vi "MainJSON.vi"(7 "Type and Defaults":variant, 8 "error in":errorcluster, 9 "pathList":string[](array[string])=["$.AnalyticsParameters"], 10 "basePath in":string, 11 "JSON String":string) -> (0 "error out":errorcluster, 1 "Oveerride JSON DATATYPE":T1, 2 "Error Message":string, 3 "VClusterOut":variant)   [LabVIEW 2015, in "Zen Analytics.lvclass"]
doc: "The input array of strings represent the <b>JSON paths</b> to specific elements in the JSON string. These elements are accessed through the path input and the output is provided in the form of <b>VCluster</b> (the bundled form of the input path elements). \nFurthermore, you may use the <b>Variant to Data</b> SubVI to convert back the Variant to the required Cluster type you want."
uses:
  Zen Analytics.lvclass
  Dependency/Override JSON.ctl
  <vilib>/Utility/Data Type/Type Definitions/Data Type.ctl
  <vilib>/regexp/Match Regular Expression.xnode
  <vilib>/addons/_JKI.lib/Serialization/JSON/JKI JSON Serialization.lvlib
  <vilib>/Utility/Data Type/NI_Data Type.lvlib
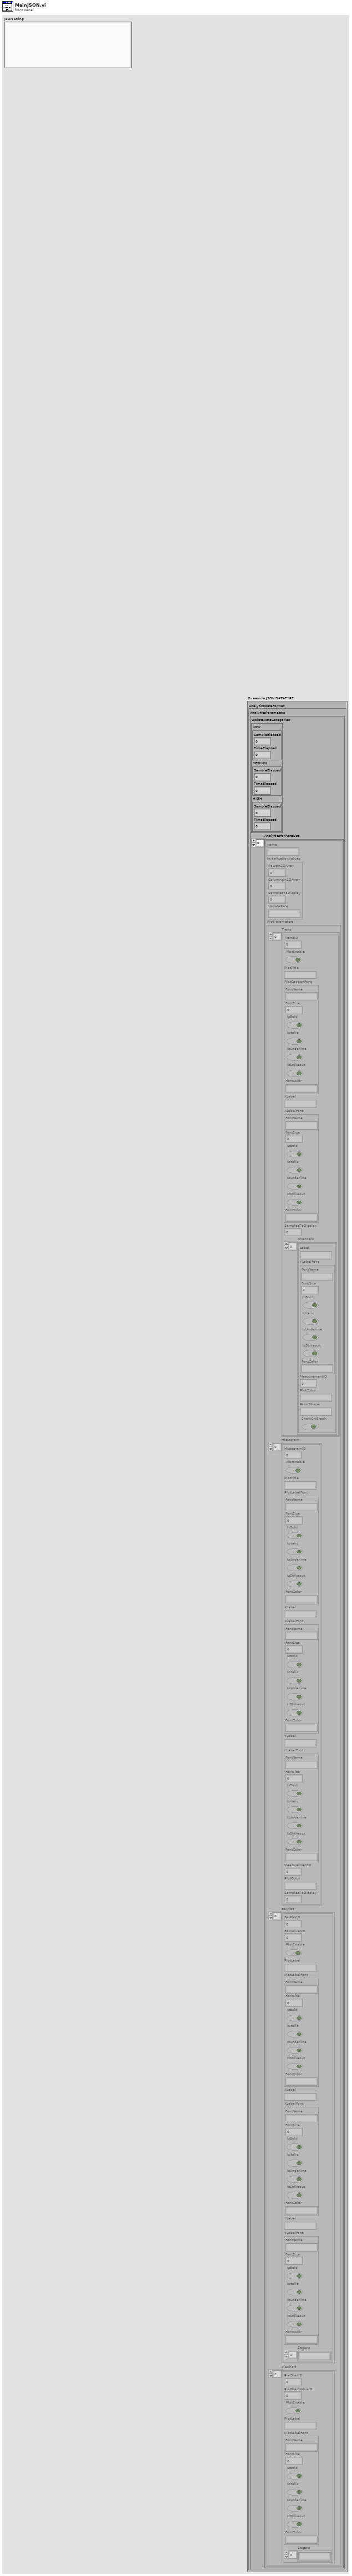
[diagram p1: front panel]
types:
  T1 = typedef "Zen Analytics.lvclass/Override JSON.ctl" = cluster{"AnalyticsDataFormat":cluster{"AnalyticsParameters":cluster{"UpdateRateCategories":cluster{"LOW":cluster{"SampleElapsed":i32, "TimeElapsed":i32}, "MEDIUM":cluster{"SampleElapsed":i32, "TimeElapsed":i32}, "HIGH":cluster{"SampleElapsed":i32, "TimeElapsed":i32}}, "AnalyticsForPartsList":cluster{"Name":string, "InitializationValues":cluster{"RowsIn2DArray":i32, "ColumnsIn2DArray":i32, "SamplesToDisplay":i32, "UpdateRate":string}, "PlotParameters":cluster{"Trend":cluster{"TrendID":i32, "PlotEnable":bool, "PlotTitle":string, "PlotCaptionFont":cluster{"FontName":string, "FontSize":i32, "IsBold":bool, "IsItalic":bool, "IsUnderline":bool, "IsStrikeout":bool, "FontColor":string}, "XLabel":string, "XLabelFont":cluster{"FontName":string, "FontSize":i32, "IsBold":bool, "IsItalic":bool, "IsUnderline":bool, "IsStrikeout":bool, "FontColor":string}, "SamplesToDisplay":i32, "Channels":cluster{"Label":string, "YLabelFont":cluster{"FontName":string, "FontSize":i32, "IsBold":bool, "IsItalic":bool, "IsUnderline":bool, "IsStrikeout":bool, "FontColor":string}, "MeasurementID":i32, "PlotColor":string, "PointShape":string, "ShowOnGraph":bool}[]}[], "Histogram":cluster{"HistogramID":i32, "PlotEnable":bool, "PlotTitle":string, "PlotLabelFont":cluster{"FontName":string, "FontSize":i32, "IsBold":bool, "IsItalic":bool, "IsUnderline":bool, "IsStrikeout":bool, "FontColor":string}, "XLabel":string, "XLabelFont":cluster{"FontName":string, "FontSize":i32, "IsBold":bool, "IsItalic":bool, "IsUnderline":bool, "IsStrikeout":bool, "FontColor":string}, "YLabel":string, "YLabelFont":cluster{"FontName":string, "FontSize":i32, "IsBold":bool, "IsItalic":bool, "IsUnderline":bool, "IsStrikeout":bool, "FontColor":string}, "MeasurementID":i32, "PlotColor":string, "SamplesToDisplay":i32}[], "BarPlot":cluster{"BarPlotID":i32, "BarValuesID":i32, "PlotEnable":bool, "PlotLabel":string, "PlotLabelFont":cluster{"FontName":string, "FontSize":i32, "IsBold":bool, "IsItalic":bool, "IsUnderline":bool, "IsStrikeout":bool, "FontColor":string}, "XLabel":string, "XLabelFont":cluster{"FontName":string, "FontSize":i32, "IsBold":bool, "IsItalic":bool, "IsUnderline":bool, "IsStrikeout":bool, "FontColor":string}, "YLabel":string, "YLabelFont":cluster{"FontName":string, "FontSize":i32, "IsBold":bool, "IsItalic":bool, "IsUnderline":bool, "IsStrikeout":bool, "FontColor":string}, "Sectors":string[]}[], "PieChart":cluster{"PieChartID":i32, "PieChartValueID":i32, "PlotEnable":bool, "PlotLabel":string, "PlotLabelFont":cluster{"FontName":string, "FontSize":i32, "IsBold":bool, "IsItalic":bool, "IsUnderline":bool, "IsStrikeout":bool, "FontColor":string}, "Sectors":string[]}[]}}[]}}}
  T2 = typedef "NI_Data Type.lvlib/Data Type.ctl" = enum8{"Invalid Type", "Void", "I8", "I16", "I32", "I64", "U8", "U16", "U32", "U64", "Single Float", "Double Float", "Extended Float", "Single Complex", "Double Complex", "Extended Complex", "Enum U8", "Enum U16", "Enum U32", "Enum U64", "Single Float With Unit", "Double Float With Unit", "Extended Float With Unit", "Single Complex with Unit", "Double Complex with Unit", "Extended Complex with Unit", "Boolean", "String", "Path", "Picture", "Tag", "Array", "Cluster", "Variant", "LV Variant", "Waveform", "Timestamp", "Digital Waveform", "Digital Data", "ExpressData", "Refnum", "External Data", "VI", "Poly VI", "LabVIEW Class Instance", "Fixed Point"}
  T3 = cluster{"AnalyticsParameters":cluster{"UpdateRateCategories":cluster{"LOW":cluster{"SampleElapsed":i32, "TimeElapsed":i32}, "MEDIUM":cluster{"SampleElapsed":i32, "TimeElapsed":i32}, "HIGH":cluster{"SampleElapsed":i32, "TimeElapsed":i32}}, "AnalyticsForPartsList":cluster{"Name":string, "InitializationValues":cluster{"RowsIn2DArray":i32, "ColumnsIn2DArray":i32, "SamplesToDisplay":i32, "UpdateRate":string}, "PlotParameters":cluster{"Trend":cluster{"TrendID":i32, "PlotEnable":bool, "PlotTitle":string, "PlotCaptionFont":cluster{"FontName":string, "FontSize":i32, "IsBold":bool, "IsItalic":bool, "IsUnderline":bool, "IsStrikeout":bool, "FontColor":string}, "XLabel":string, "XLabelFont":cluster{"FontName":string, "FontSize":i32, "IsBold":bool, "IsItalic":bool, "IsUnderline":bool, "IsStrikeout":bool, "FontColor":string}, "SamplesToDisplay":i32, "Channels":cluster{"Label":string, "YLabelFont":cluster{"FontName":string, "FontSize":i32, "IsBold":bool, "IsItalic":bool, "IsUnderline":bool, "IsStrikeout":bool, "FontColor":string}, "MeasurementID":i32, "PlotColor":string, "PointShape":string, "ShowOnGraph":bool}[]}[], "Histogram":cluster{"HistogramID":i32, "PlotEnable":bool, "PlotTitle":string, "PlotLabelFont":cluster{"FontName":string, "FontSize":i32, "IsBold":bool, "IsItalic":bool, "IsUnderline":bool, "IsStrikeout":bool, "FontColor":string}, "XLabel":string, "XLabelFont":cluster{"FontName":string, "FontSize":i32, "IsBold":bool, "IsItalic":bool, "IsUnderline":bool, "IsStrikeout":bool, "FontColor":string}, "YLabel":string, "YLabelFont":cluster{"FontName":string, "FontSize":i32, "IsBold":bool, "IsItalic":bool, "IsUnderline":bool, "IsStrikeout":bool, "FontColor":string}, "MeasurementID":i32, "PlotColor":string, "SamplesToDisplay":i32}[], "BarPlot":cluster{"BarPlotID":i32, "BarValuesID":i32, "PlotEnable":bool, "PlotLabel":string, "PlotLabelFont":cluster{"FontName":string, "FontSize":i32, "IsBold":bool, "IsItalic":bool, "IsUnderline":bool, "IsStrikeout":bool, "FontColor":string}, "XLabel":string, "XLabelFont":cluster{"FontName":string, "FontSize":i32, "IsBold":bool, "IsItalic":bool, "IsUnderline":bool, "IsStrikeout":bool, "FontColor":string}, "YLabel":string, "YLabelFont":cluster{"FontName":string, "FontSize":i32, "IsBold":bool, "IsItalic":bool, "IsUnderline":bool, "IsStrikeout":bool, "FontColor":string}, "Sectors":string[]}[], "PieChart":cluster{"PieChartID":i32, "PieChartValueID":i32, "PlotEnable":bool, "PlotLabel":string, "PlotLabelFont":cluster{"FontName":string, "FontSize":i32, "IsBold":bool, "IsItalic":bool, "IsUnderline":bool, "IsStrikeout":bool, "FontColor":string}, "Sectors":string[]}[]}}[]}}
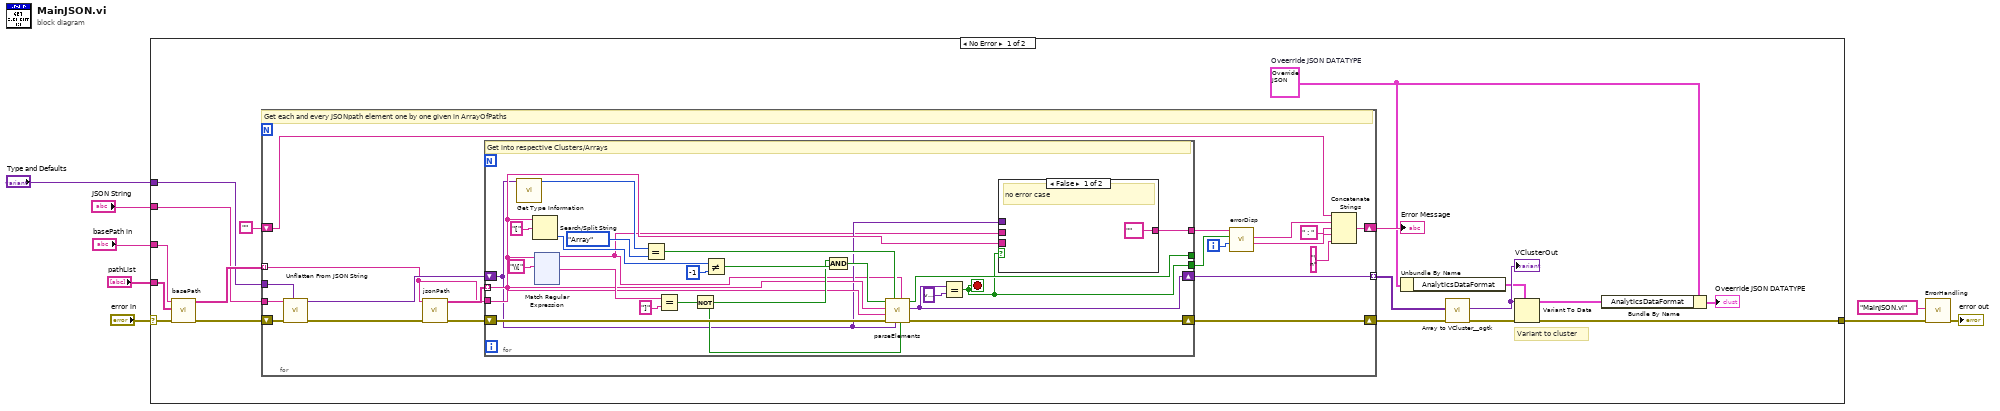
[diagram p0: block diagram]
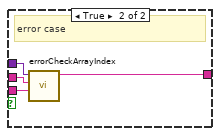
[diagram p2: hidden frame]
diagram:
  n1 = case shown="No Error" "error in" {
    selector: "error in" -> [w24 w189]
    tunnel: [w13 w189] -> w8
    tunnel: "Type and Defaults" -> [w21 _]
    tunnel: "basePath in" -> [w20 _]
    tunnel: "JSON String" -> [w19 _]
    tunnel: "pathList" -> [w18 _]
    frame No Error {
      w11 = T1 {"AnalyticsDataFormat"={"AnalyticsParameters"={"UpdateRateCategories"={"LOW"={"SampleElapsed"=0, "TimeElapsed"=0}, "MEDIUM"={"SampleElapsed"=0, "TimeElapsed"=0}, "HIGH"={"SampleElapsed"=0, "TimeElapsed"=0}}, "AnalyticsForPartsList"=[]}}}  # Oveerride JSON DATATYPE
      # "Variant to cluster"
      n2 = call "basePath.vi"("error in (no error)"=w24, "pathList"=w18, "basePath in"=w20) -> ("error out"=w23:errorcluster, "pathArray out"=w22:string[])  [unwired: 7 in]
      n3 = for {
        tunnel: w22 -> [w39] mode=indexing
        tunnel: w19 -> [w45]
        shift-right: [w40] -> w26
        shift-left: w23 -> [w44]
        tunnel: [w35] -> w25 mode=indexing
        tunnel: w21 -> [w38]
        shift-right: [w28] -> w17
        shift-left: "" -> [w27]
        i -> [w37]
        # "Get each and every JSONpath element one by one given in ArrayOfPaths"
        n4 = call <vilib>:"Unflatten From JSON String.vi"("Type and Defaults"=w38, "error in (no error)"=w44, "JSON String"=w45) -> ("error out"=w36:errorcluster, "Variant"=w43:variant)  [unwired: 7 in]
        n5 = call "jsonPath.vi"("error in (no error)"=w36, "json path in"=w39) -> ("error out"=w41:errorcluster, "output array of keys"=w42:string[])  [unwired: 8 in]
        n6 = for {
          tunnel: w42 -> [w50] mode=indexing
          shift-right: [w52] -> w35
          shift-left: w43 -> [w49]
          shift-right: [w67] -> w40
          shift-left: w41 -> [w68]
          tunnel: w39 -> [w54]
          tunnel: [w47] -> _
          tunnel: [w46] -> w34
          tunnel: [w51] -> w33
          stop <- w46 stop-if-true
          # "Get into respective Clusters/Arrays"
          n7 = call <vilib>:"Get Type Information.vi"("Variant"=w49) -> ("Type"=w57:T2)  [unwired: 6 in, 4 out]
          n8 = Search/Split String(string=w50, search string/char (-)="[") -> (offset of match=w64:i32)  [unwired: 1 in, 2 out]
          n9 = xnode "Match Regular Expression"("input string"=w50, "regular expression"="\\[") -> ("before match"=w48:string, "after match"=w62:string)  [unwired: 4 in, 3 out]
          n10 = Equal?(x=w57, y=Data_Type."Array") -> (x = y?=w55:bool)
          n11 = Equal?(x=w62, y="]") -> (x = y?=w61:bool)
          n12 = Not(x=w61) -> (.not. x?=w58:bool)
          n13 = Not Equal?(x=w64, y=-1) -> (x != y?=w60:bool)
          n14 = And(x=w58, y=w60) -> (x .and. y?=w59:bool)
          n15 = call "parseElements.vi"("<\"[]\" not present>"=w58, "requiredObjectFromPath"=w48, "Variant"=w49, "checkEmptyArrayIndices"=w55, "error in (no error)"=w68, "jsonString"=w54, "singlePathElement"=w50, "checkArraysOrClusters"=w59) -> ("error out"=w67:errorcluster, "VArray"=w52:variant, "error?"=w47:bool)  [unwired: 1 in]
          n16 = Equal?(x=w52, y=variant) -> (x = y?=w46:bool)
          n17 = case shown="False" w46 {
            tunnel: ["" ("value") w74] -> w51
            tunnel: w50 -> [_ w73]
            tunnel: w49 -> [_ w72]
            tunnel: w48 -> [_ w71]
            frame False {
              # "no error case"
            }
            frame True {
              # "error case"
              n18 = call "errorCheckArrayIndex.vi"("<single path ele>"=w73, "<req. obj>"=w71, "Variant"=w72) -> ("value"=w74:string)  [unwired: 8 in]
            }
          }
        }
        n19 = call "errorDisp.vi"("error path index in"=w37, "error?"=w34, "string check in"=w33) -> ("string check"=w31:string, "path index"=w32:string)  [unwired: 6 in, 1 out]
        n20 = Concatenate Strings(w27, w32, " : " ("string"), w31, "\n" ("string")) -> (w28:string)
      }
      "Error Message" <- w17
      n21 = Unbundle By Name(w11) -> ("AnalyticsDataFormat"=w12:T3)
      n22 = call <userlib>:"Array to VCluster__ogtk.vi"("error in (no error)"=w26, "Array"=w25) -> ("error out"=w14:errorcluster, "VCluster"=w15:variant)  [unwired: 8 in]
      "VClusterOut" <- w15
      n23 = Variant To Data(error in=w14, type=w12, Variant=w15) -> (data=w10:T3, error out=w13:errorcluster)
      n24 = Bundle By Name(cluster=w11, "AnalyticsDataFormat"=w10) -> (→"Oveerride JSON DATATYPE":T1)
    }
    frame Error {
    }
  }
  n25 = call "ErrorHandling.vi"("error in (no error)"=w8, "Vi-name"="MainJSON.vi") -> ("error out"=→"error out":errorcluster)  [unwired: 9 in]
